vi "GV-Layer-GT-zero.vi"(2 "Layer":i32) -> (7 ">0 ?":bool)   [LabVIEW 2020, in "Sgraph_lib_V1.lvlib" / "Gviewer.lvclass"]
doc: "Layer compare > 0 ?\n\n(also if layer is negative due to disk usage)"
uses:
  Gviewer.lvclass
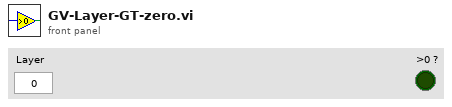
[diagram p1: front panel]
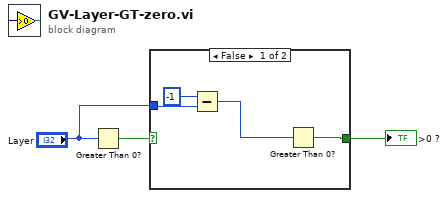
[diagram p0: block diagram]
diagram:
  n1 = Greater Than 0?(x="Layer") -> (x > 0?=w3:bool)
  n2 = case shown="False" w3 {
    selector: w3 -> [_ w8]
    tunnel: [w4 w8] -> w2
    tunnel: "Layer" -> [w7 _]
    frame False {
      n3 = Subtract(x=-1, y=w7) -> (x-y=w5:i32)
      n4 = Greater Than 0?(x=w5) -> (x > 0?=w4:bool)
    }
    frame True {
    }
  }
  ">0 ?" <- w2
